vi "get_settings_cluster.vi"(8 "error in (no error)":errorcluster, 11 "TrajectoryAK101022Resonance in":refnum<class "TrajectoryAK101022Resonance.lvclass">) -> (0 "error out":errorcluster, 2 "settings cluster (variant)":variant, 3 "TrajectoryAK101022Resonance out":refnum<class "TrajectoryAK101022Resonance.lvclass">)   [LabVIEW 2010, in "TrajectoryAK101022Resonance.lvclass"]
uses:
  TrajectoryAK101022Resonance.lvclass
  TrajectoryAK101022Resonance.lvclass/TrajectoryAK101022Resonance.ctl
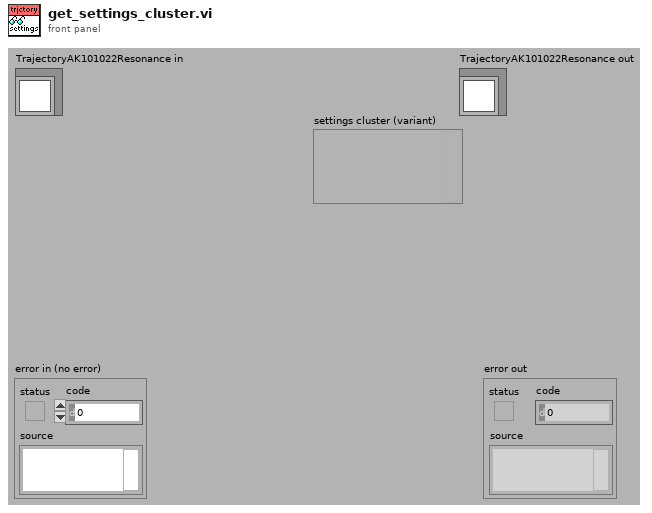
[diagram p1: front panel]
types:
  T1 = typedef "TrajectoryAK101022Resonance.lvclass/settings_cluster.ctl" = cluster{"x resolution":i32, "x offset flyforward fraction":dbl, "x offset flyback fraction":dbl, "x scan segment fraction":dbl, "zoom":dbl, "level High":dbl, "phase":dbl, "lines per z step":i32, "level undershoot":dbl, "level overshoot":dbl, "samples level high":u16, "samples overshoot":u16, "samples ramp":u16, "samples undershoot":u16, "filter order":u16, "high filter cutoff":dbl, "low filter cutoff":dbl, "filtertype":enum16{"Lowpass", "Highpass", "Bandpass", "Bandstop"}, "x amplitude":u16, "y resolution (nr. of lines)":i32, "y step size":u16, "iterations per pixel":u16, "number of frames":i32, "y offset (pixels)":u16, "z step size":dbl[unit], "repetitions (volumes or planes)":i32, "z-function-type":enum16{"Sine", "Stack", "Step"}, "bi-directional?":bool, "phase":dbl[unit], "z-amplitude(sine)":dbl[unit], "angle fraction (sine)":dbl, "ETL phase delay":dbl[unit], "ETL amplitude conversion":dbl[unit], "number of z/intensity tupels":i32}
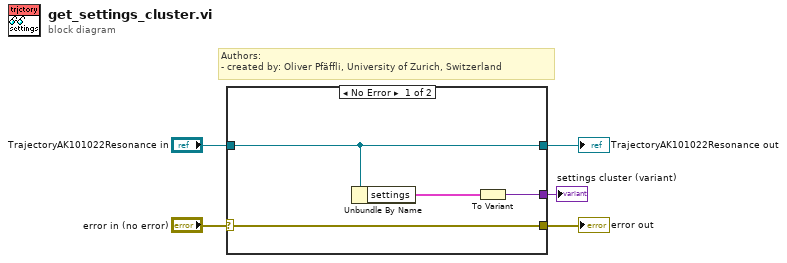
[diagram p0: block diagram]
diagram:
  # "Authors: \n- created by: Oliver Pfäffli, University of Zurich, Switzerland"
  n1 = case shown="No Error" "error in (no error)" {
    selector: "error in (no error)" -> [w9 w11]
    tunnel: [w9 w11] -> w4
    tunnel: [w8 w10] -> w2
    tunnel: "TrajectoryAK101022Resonance in" -> [w8 w10]
    tunnel: [w6 _] -> w1
    frame No Error {
      n2 = Unbundle By Name(w8) -> ("settings"=w7:T1)
      n3 = To Variant(anything=w7) -> (Variant=w6:variant)
    }
    frame Error {
    }
  }
  "error out" <- w4
  "TrajectoryAK101022Resonance out" <- w2
  "settings cluster (variant)" <- w1
